vi "APS get board param.vi"(8 "error in (no error)":errorcluster caption="错误输入（无错误）", 9 "BOD_Param":i32, 10 "BOD_Param_No":i32, 11 "Board_ID":i32) -> (0 "error out":errorcluster caption="错误输出", 1 "BOD_Param out":i32, 3 "function return":i32)   [LabVIEW 2011, in "APS168.lvlib"]
doc: "I32 FNTYPE APS_get_board_param( I32 Board_ID, I32 BOD_Param_No, I32 *BOD_Param );"
uses:
  APS168.lvlib
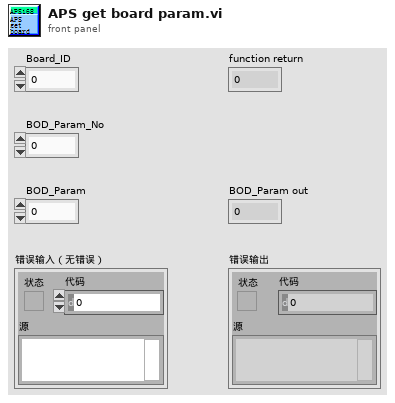
[diagram p1: front panel]
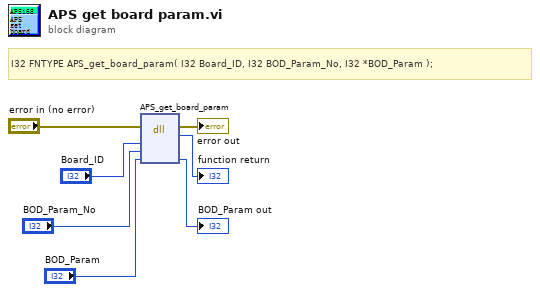
[diagram p0: block diagram]
diagram:
  # "I32 FNTYPE APS_get_board_param( I32 Board_ID, I32 BOD_Param_No, I32 *BOD_Param );"
  n1 = dll-call lib="PTH1Labs E软件ADLINK 204CAPS_1_7_1_LIB line 连续运动204APS168.*" fn="APS_get_board_param"(error in="error in (no error)", "Board_ID"="Board_ID", "BOD_Param_No"="BOD_Param_No", "BOD_Param"="BOD_Param") -> (error out=→"error out":errorcluster, →"function return":i32, "BOD_Param"=→"BOD_Param out":i32)  [unwired: 4 in, 1 out]
